vi "ex1.1.vi"() -> ()   [LabVIEW 2022 SP3]
uses:
  <vilib>/numeric/Random Number (Range) I64.vi
  7323c38f-d153-4936-93a6-4a742cffa189.vi
  <vilib>/numeric/sub_Random U32.vi
  <vilib>/Array/Sort 2D Array - Pop Stack.vi
  <vilib>/Array/Sort 2D Array - Push Stack.vi
  7323c38f-d153-4936-93a6-4a742cffa189.vi/269d4b3b-47f5-49e3-8884-44851e4dd9d5.vi
  7323c38f-d153-4936-93a6-4a742cffa189.vi/6d99389c-673d-4efb-bf33-19b32bcf4cf8.vi
panel:
  out "sorted 2D array":i64[][](array[numeric])
  in  "Sort By:":enum16{"column", "row"}(ring)
  in  "Select Column":dbl
  in  "Select Row":dbl
  in  "Numeric":i32
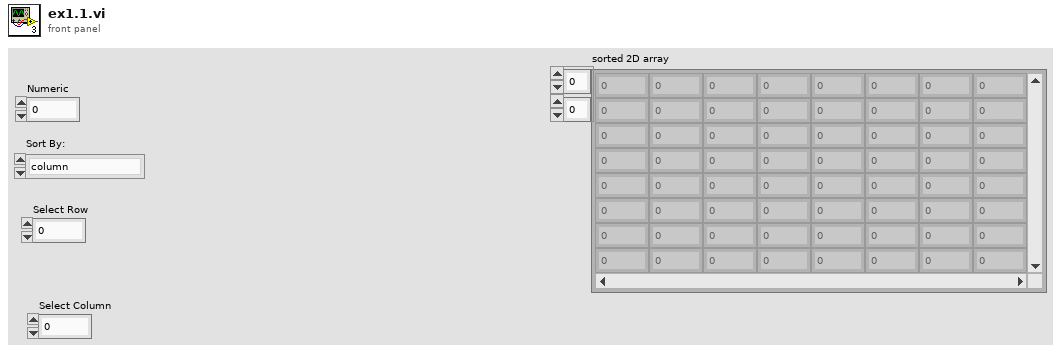
[diagram p1: front panel]
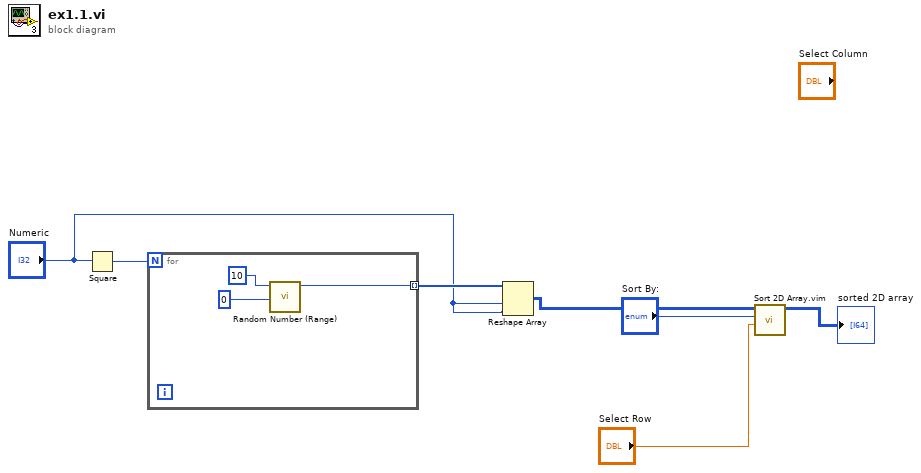
[diagram p0: block diagram]
diagram:
  n1 = Square(x="Numeric") -> (x^2=w5:i32)
  n2 = for {
    N: w5 -> [_]
    tunnel: [w10] -> w7 mode=indexing
    n3 = call-poly <vilib>:"Random Number (Range).vi"("lower bound (-100)"=i64 0, "upper bound (100)"=i64 10) -> ("number"=w10:i64)  [unwired: 9 in]
  }
  n4 = Reshape Array(w7, "Numeric", "Numeric") -> (w3:i64[][])
  n5 = call "Sort 2D Array.vim"("index"="Select Row", "dimension to index (column)"="Sort By:", "2D array"=w3) -> ("sorted 2D array"=→"sorted 2D array":i64[][])  [unwired: 7 in, 1 out]
